vi "ExecEng_ImportSequenceFromFile.vi"(8 "error in (no error)":errorcluster, 11 "VI Server.RefsCluster in":T1) -> (0 "error out":errorcluster, 3 "VI Server.RefsCluster out":T1)   [LabVIEW 2020]
uses:
  LabVIEW 2020 Toolkits/VI Server Toolkit/VI Server_TypeDefs/VI Server_RefsCluster.ctl
  LabVIEW 2020 Toolkits/toolkits_lv2020_32bit/Synchronization.llb/SynchRefs_SetGet.ctl
panel:
  in  "SourceFileFolder":path
  in  "ArbitraryFileSelector":path caption="Arbitrary File Selector"
  in  "SourceFile":u16(ring) caption="Source File" items=["Instrument Sequence", "Arbitrary File"]
  in  "Sequence.InsertAfterSelection":bool
  in  "Sequence.InsertBeforeSelection":bool
  in  "Sequence.InsertAtBottom":bool
  in  "Sequence.InsertAtTop":bool
  in  "EXIT":bool
  in  "SequenceFile.Open":bool
  in  "TestCaseConfiguration":i32[](listbox) caption="Test Case Configuration"
  in  "Sequence.FileNames":u16(ring) caption="Sequence File Names:"
  in  "SequenceFile.Path":path[](array[path])
  # "IMPORT SEQUENCE FROM FILE"
  # "M"
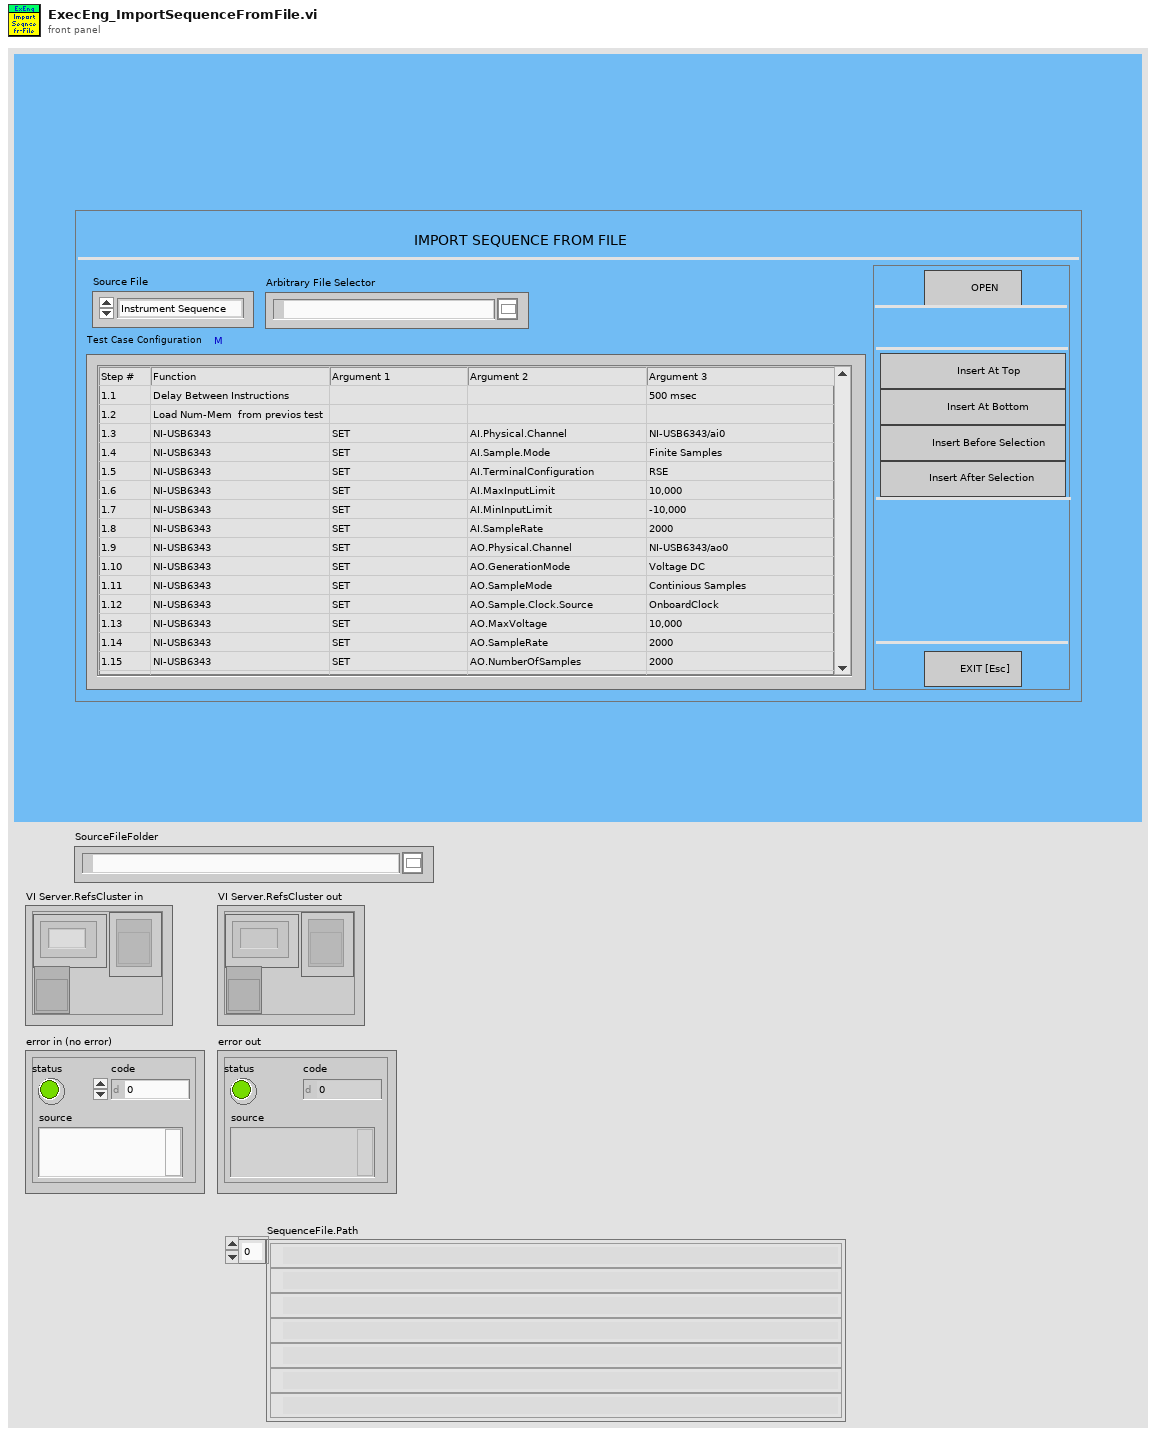
[diagram p1: front panel]
types:
  T1 = typedef "VI Server_RefsCluster.ctl" = cluster{"Labels":string[], "Refs":refnum<vi>[], "VI Ref":refnum<vi>}
  T2 = typedef "SynchRefs_SetGet.ctl" = enum16{"Set", "Get"}
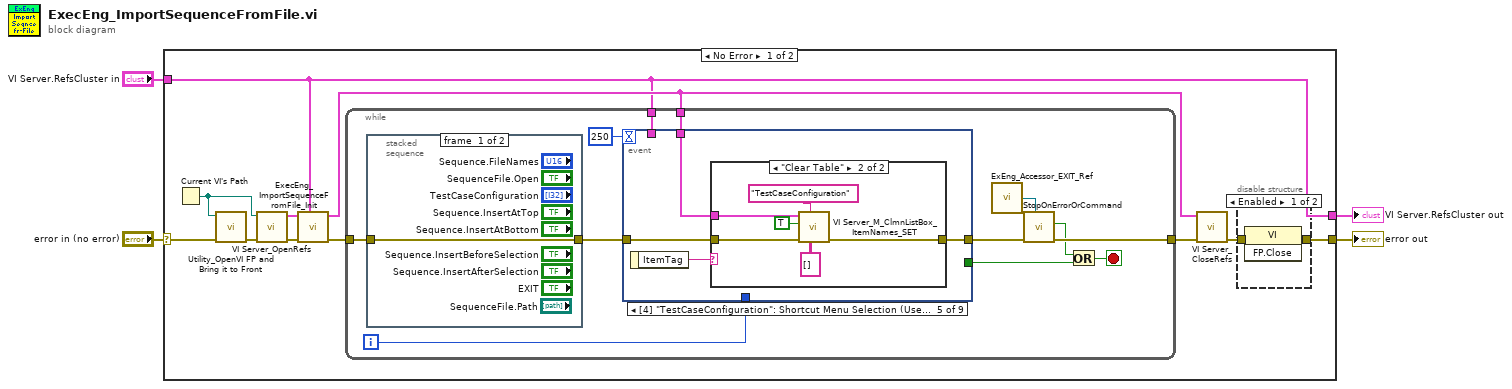
[diagram p0: block diagram]
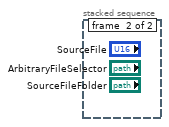
[diagram p3: hidden frame]
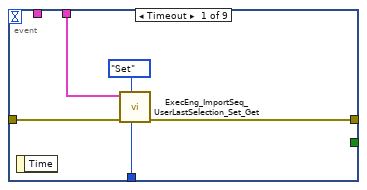
[diagram p4: hidden frame]
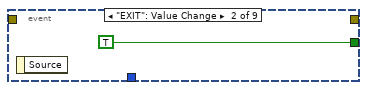
[diagram p5: hidden frame]
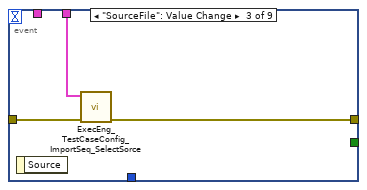
[diagram p6: hidden frame]
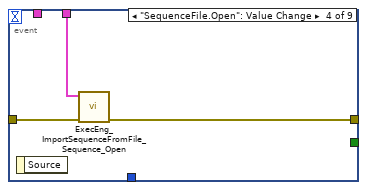
[diagram p7: hidden frame]
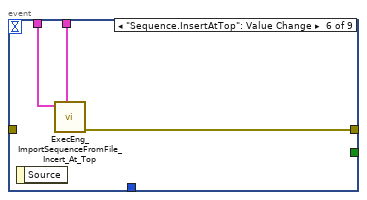
[diagram p9: hidden frame]
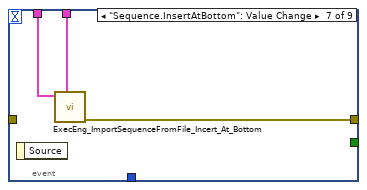
[diagram p10: hidden frame]
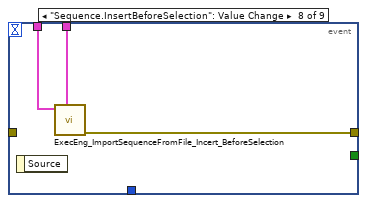
[diagram p11: hidden frame]
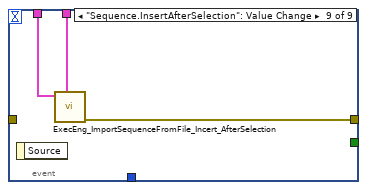
[diagram p12: hidden frame]
diagram:
  n1 = case shown="No Error" "error in (no error)" {
    selector: "error in (no error)" -> [w14 w67]
    tunnel: "VI Server.RefsCluster in" -> [w5 _]
    tunnel: [w8 w67] -> w1
    tunnel: [w5 _] -> w4
    frame No Error {
      n2 = Current VI's Path() -> (path=w6:path)
      n3 = call "Utility_OpenVI FP and Bring it to Front.vi"("error in (no error)"=w14, "VI Path"=w6) -> ("error out"=w13:errorcluster)  [unwired: 9 in]
      n4 = call "VI Server_OpenRefs.vi"("error in"=w13, "VI Path"=w6) -> ("error out"=w12:errorcluster, "VI Server.RefsCluster"=w10:T1)  [unwired: 8 in]
      n5 = call "ExecEng_ImportSequenceFromFile_Init.vi"("VI Server.RefsCluster.TopVI"=w5, "error in (no error)"=w12, "VI Server.RefsCluster.Local"=w10) -> ("error out"=w15:errorcluster, "VI Server.RefsCluster.DUP"=w7:T1)  [unwired: 7 in]
      n6 = while {
        tunnel: w15 -> [w30]
        tunnel: [w26] -> w11
        tunnel: w7 -> [w22]
        tunnel: w5 -> [w21]
        i -> [w19]
        stop <- w23 stop-if-true
        n7 = stacked-sequence {
          tunnel: w30 -> [w31 _]
          tunnel: [w31 _] -> w20
          frame #0 {
          }
          frame #1 {
          }
        }
        n8 = event shown="[4] \"TestCaseConfiguration\": Shortcut Menu Selection (User)" {
          selector: _ -> [_ _ _ _ _ _ _ _ _]
          dyn-events: _ -> [_ _ _ _ _ _ _ _ _]
          timeout: 250 -> [_ _ _ _ _ _ _ _ _]
          tunnel: [w36 _ w38 w43 w45 w57 w58 w63 w66] -> w27
          tunnel: [_ TRUE _ _ _ _ _ _ _] -> w24
          tunnel: w22 -> [w34 _ w39 w42 w44 w55 w59 w61 w64]
          tunnel: w21 -> [_ _ _ _ _ w56 w60 w62 w65]
          tunnel: w20 -> [w35 _ w40 w41 w46 _ _ _ _]
          tunnel: w19 -> [w32 _ _ _ _ _ _ _ _]
          event Timeout {
            n9 = event-data() -> ()  [unwired: 1 in, 1 out]
            n10 = call "ExecEng_ImportSeq_UserLastSelection_Set_Get.vi"("LoopCounter"=w32, "SynchRefs.Set/Get"=SynchRefs_SetGet."Set", "error in"=w35, "VI Server.RefsCluster"=w34) -> ("error out"=w36:errorcluster)  [unwired: 6 in, 1 out]
          }
          event "EXIT": Value Change {
            n11 = event-data() -> ()  [unwired: 1 in, 1 out]
          }
          event "SourceFile": Value Change {
            n12 = event-data() -> ()  [unwired: 1 in, 1 out]
            n13 = call "ExecEng_TestCaseConfig_ImportSeq_SelectSorce.vi"("error in (no error)"=w40, "VI Server.RefsCluster"=w39) -> ("error out"=w38:errorcluster)  [unwired: 9 in]
          }
          event "SequenceFile.Open": Value Change {
            n14 = event-data() -> ()  [unwired: 1 in, 1 out]
            n15 = call "ExecEng_ImportSequenceFromFile_Sequence_Open.vi"("error in (no error)"=w41, "VI Server Cluster"=w42) -> ("error out"=w43:errorcluster)  [unwired: 9 in]
          }
          event "TestCaseConfiguration": Shortcut Menu Selection (User) {
            n16 = event-data() -> ("ItemTag"=w47:string)  [unwired: 1 in]
            n17 = case shown="\"Clear Table\"" w47 {
              tunnel: w46 -> [w48 w54]
              tunnel: [w48 w53] -> w45
              tunnel: w44 -> [_ w51]
              frame "False", Default {
              }
              frame "Clear Table" {
                n18 = call "VI Server_M_ClmnListBox_ItemNames_SET.vi"("Item Names"=string[][] [], "Label"="TestCaseConfiguration", "error in"=w54, "SingleInstance"=TRUE, "VI Server.RefsCluster"=w51) -> ("error out"=w53:errorcluster)  [unwired: 4 in, 2 out]
              }
            }
          }
          event "Sequence.InsertAtTop": Value Change {
            n19 = event-data() -> ()  [unwired: 1 in, 1 out]
            n20 = call "ExecEng_ImportSequenceFromFile_Incert_At_Top.vi"("VI Server.RefsCluster(Local)"=w55, "VI Server.RefsCluster(TopLevel)"=w56) -> ("error out"=w57:errorcluster)  [unwired: 9 in]
          }
          event "Sequence.InsertAtBottom": Value Change {
            n21 = event-data() -> ()  [unwired: 1 in, 1 out]
            n22 = call "ExecEng_ImportSequenceFromFile_Incert_At_Bottom.vi"("VI Server.RefsCluster(Local)"=w59, "VI Server.RefsCluster(TopLevel)"=w60) -> ("error out"=w58:errorcluster)  [unwired: 9 in]
          }
          event "Sequence.InsertBeforeSelection": Value Change {
            n23 = event-data() -> ()  [unwired: 1 in, 1 out]
            n24 = call "ExecEng_ImportSequenceFromFile_Incert_BeforeSelection.vi"("VI Server.RefsCluster(Local)"=w61, "VI Server.RefsCluster(TopLevel)"=w62) -> ("error out"=w63:errorcluster)  [unwired: 9 in]
          }
          event "Sequence.InsertAfterSelection": Value Change {
            n25 = event-data() -> ()  [unwired: 1 in, 1 out]
            n26 = call "ExecEng_ImportSequenceFromFile_Incert_AfterSelection.vi"("VI Server.RefsCluster(Local)"=w64, "VI Server.RefsCluster(TopLevel)"=w65) -> ("error out"=w66:errorcluster)  [unwired: 9 in]
          }
        }
        n27 = call "ExEng_Accessor_EXIT_Ref.vi"() -> ("EXIT"=w28:refnum<notifier>)  [unwired: 6 in]
        n28 = call "StopOnErrorOrCommand.vi"("STOP"=w28, "error in (no error)"=w27) -> ("error out"=w26:errorcluster, "STOP"=w25:bool)  [unwired: 8 in]
        n29 = Or(x=w25, y=w24) -> (x .or. y?=w23:bool)
      }
      n30 = call "VI Server_CloseRefs.vi"("error in"=w11, "VI Server.RefsCluster"=w7) -> ("error out"=w9:errorcluster)  [unwired: 9 in]
      n31 = disable-structure shown="Enabled" {
        disable-tunnel: w9 -> [w17 w18]
        disable-tunnel: [w16 w18] -> w8
        frame Enabled {
          n32 = invoke class="VI" method="FP.Close"(error in=w17) -> (error out=w16:errorcluster)  [unwired: 2 in, 2 out]
        }
        frame Disabled {
        }
      }
    }
    frame Error {
    }
  }
  "VI Server.RefsCluster out" <- w4
  "error out" <- w1
